vi "Auto_Find.vi"(0 "Start WL -- nm":dbl=1530.0 format="%.2f", 1 "Type of Measurement":u16(ring)=1 items=["Reflection", "Transmission"], 5 "End WL -- nm":dbl=1550.0 format="%.2f", 7 "ampSize (32768)":i32=131072, 9 "Auto-Find Type":enum8{"Bandstop - amp", "Bandpass - phase"}(ring), 11 "error in (no error)":errorcluster) -> (4 "Length of DUT (m)":dbl format="%.3f", 8 "dutIndex":u32, 15 "error out":errorcluster)   [LabVIEW 2024]
uses:
  OVA32.dll
panel:
  out "Output Array":dbl[](graph)
  # "DUT Length Finder Utility"
  # "=>"
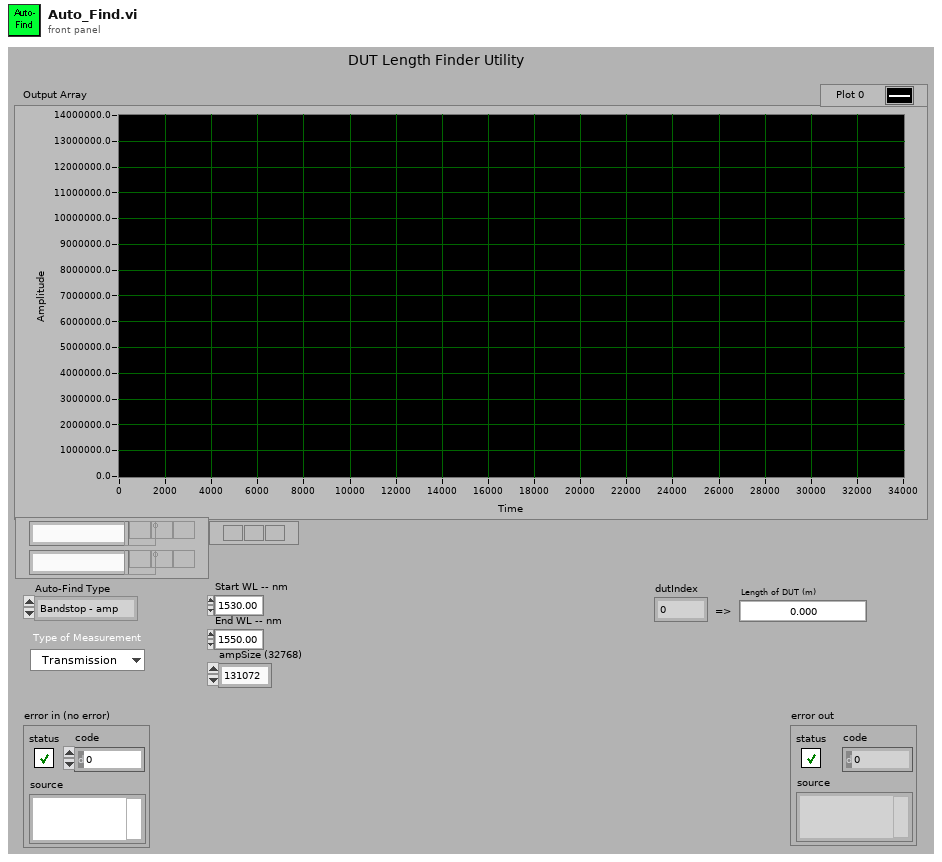
[diagram p1: front panel]
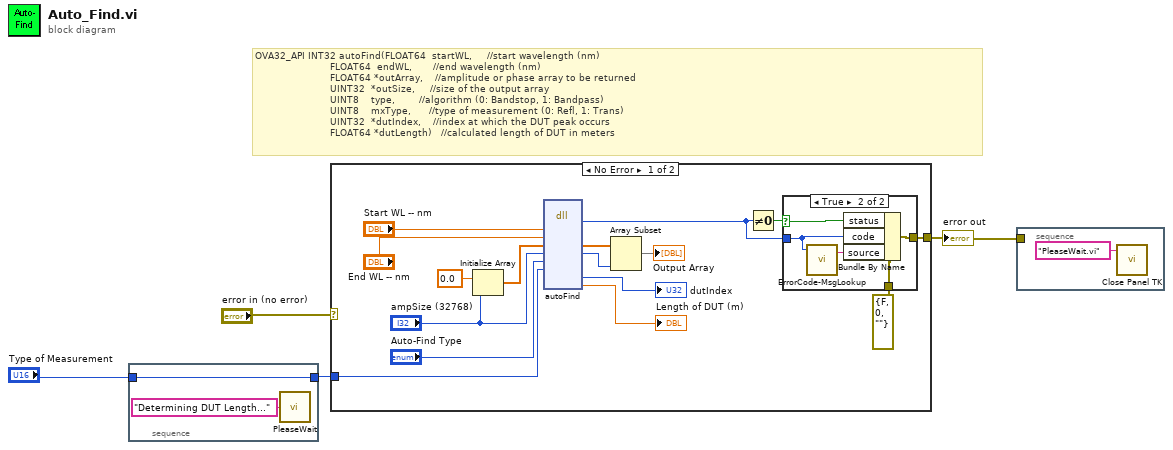
[diagram p0: block diagram]
diagram:
  # "OVA32_API INT32 autoFind(FLOAT64  startWL,     //start wavelength (nm)\n                         FLOAT64  endWL,       //end wavelength (nm)\n                         FLOAT64 *outArray,    //amplitude or phase array to be returned   \n                         UINT32  *outSize,     //size of the output array\n                         UINT8    type,        //algorithm (0: Bandstop, 1: Bandpass)\n                         UINT8    mxType,      //type of measurement (0: Refl, 1: Trans)\n                         UINT32  *dutIndex,    //index at which the DUT peak occurs\n                         FLOAT64 *dutLength)   //calculated length of DUT in meters"
  n1 = stacked-sequence {
    tunnel: [w6] -> w2
    tunnel: "Type of Measurement" -> [w6]
    frame #0 {
      n2 = call "PleaseWait.vi"("Current Test 2"="Determining DUT Length..." ("Current Test")) -> ()  [unwired: 1 in]
    }
  }
  n3 = case shown="No Error" "error in (no error)" {
    selector: "error in (no error)" -> [_ w29]
    tunnel: [w20 w29] -> w4
    tunnel: w2 -> [w13 _]
    frame No Error {
      n4 = Initialize Array(0.0 ("Element Data"), "ampSize (32768)") -> (w15:dbl[])
      n5 = dll-call lib="OVA32.dll" fn="autoFind"("startWL"="Start WL -- nm", "endWL"="End WL -- nm", "outArray"=w15, "outSize"="ampSize (32768)", "method"="Auto-Find Type", "mxType"=w13) -> ("return type"=w17:i32, "outArray"=w9:dbl[], "outSize"=w7:u32, "dutIndex"=→"dutIndex":u32, "dutLength"=→"Length of DUT (m)":dbl)  [unwired: 9 in, 2 out]
      n6 = Array Subset(array=w9, length=w7) -> (→"Output Array":dbl[])  [unwired: 1 in]
      n7 = Not Equal To 0?(x=w17) -> (x != 0?=w21:bool)
      n8 = case shown="True" w21 {
        selector: w21 -> [_ w26]
        tunnel: w17 -> [_ w25]
        tunnel: [w23 w27] -> w20
        tunnel: errorcluster {"status"=FALSE, "code"=0, "source"=""} ("error out") -> [w23 w24]
        frame False {
        }
        frame True {
          n9 = call "ErrorCode-MsgLookup.vi"("DLL Return Code"=w25) -> ("Error String"=w28:string)  [unwired: 2 in, 2 out]
          n10 = Bundle By Name(cluster=w24, "status"=w26, "code"=w25, "source"=w28) -> (w27:errorcluster)
        }
      }
    }
    frame Error {
    }
  }
  "error out" <- w4
  n11 = stacked-sequence {
    tunnel: w4 -> [_]
    frame #0 {
      n12 = call "Close Panel TK.vi"("VI name"="PleaseWait.vi") -> ()  [unwired: 10 in, 1 out]
    }
  }
